vi "CheckSpeedTol (SubVI).vi"(8 "error in (no error)":errorcluster, 10 "Target Speed":sgl, 11 "Actual Speed":dbl) -> (0 "error out (no error)":errorcluster, 3 "Speed in Range?":bool)   [LabVIEW 2020]
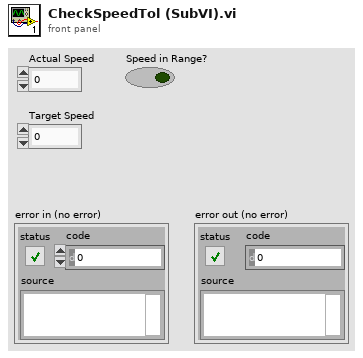
[diagram p1: front panel]
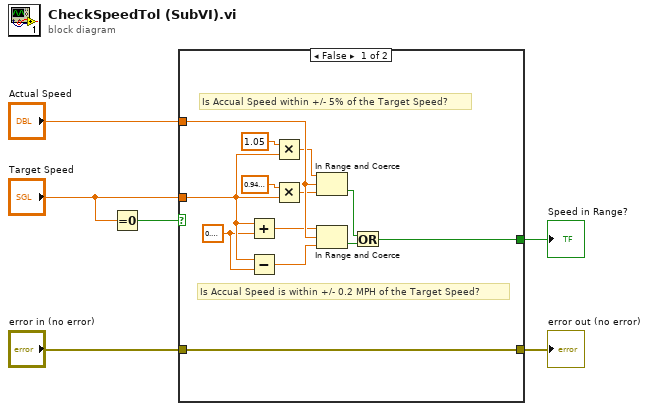
[diagram p0: block diagram]
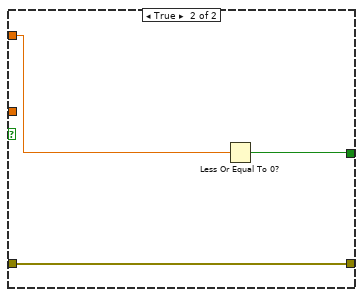
[diagram p2: hidden frame]
diagram:
  n1 = Equal To 0?(x="Target Speed") -> (x = 0?=w4:bool)
  n2 = case shown="False" w4 {
    tunnel: [w19 w22] -> w6
    tunnel: "Actual Speed" -> [w16 w20]
    tunnel: "Target Speed" -> [w14 _]
    tunnel: "error in (no error)" -> [w7 w21]
    tunnel: [w7 w21] -> w1
    frame False {
      w8 = sgl 0.2 ("y")
      # "Is Accual Speed within +/- 5% of the Target Speed?"
      # "Is Accual Speed is within +/- 0.2 MPH of the Target Speed?"
      n3 = Add(x=w14, y=w8) -> (x+y=w9:sgl)
      n4 = Subtract(x=w14, y=w8) -> (x-y=w10:sgl)
      n5 = Multiply(x=1.05, y=w14) -> (x*y=w15:dbl)
      n6 = Multiply(x=sgl 0.95, y=w14) -> (x*y=w12:sgl)
      n7 = In Range and Coerce(upper limit=w15, x=w16, lower limit=w12) -> (In Range?=w17:bool)  [unwired: 1 out]
      n8 = In Range and Coerce(upper limit=w9, x=w16, lower limit=w10) -> (In Range?=w18:bool)  [unwired: 1 out]
      n9 = Or(x=w17, y=w18) -> (x .or. y?=w19:bool)
    }
    frame True {
      n10 = Less Or Equal To 0?(x=w20) -> (x <= 0?=w22:bool)
    }
  }
  "Speed in Range?" <- w6
  "error out (no error)" <- w1
